vi "Rangel Limit.vi"(2 "Limit":dbl, 3 "Input":dbl) -> (1 "Output":dbl)   [LabVIEW 2013]
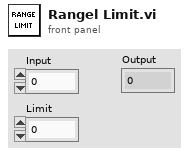
[diagram p1: front panel]
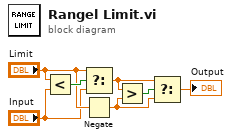
[diagram p0: block diagram]
diagram:
  n1 = Less?(x="Limit", y="Input") -> (x < y?=w7:bool)
  n2 = Select(t="Limit", s=w7, f="Input") -> (s? t:f=w3:dbl)
  n3 = Negate(x="Limit") -> (-x=w5:dbl)
  n4 = Greater?(x=w3, y=w5) -> (0:w6:bool)
  n5 = Select(t=w3, s=w6, f=w5) -> (s? t:f=→"Output":dbl)
